vi "Delete Zero.vi"(1 "Unique P-Waves":dbl[](array[numeric])) -> (0 "P-Waves Locations (s)":dbl[](array[numeric]) format="%.2p")   [LabVIEW 2018]
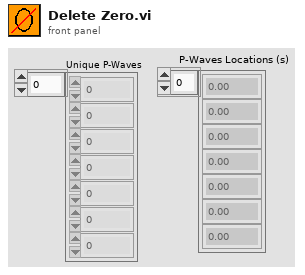
[diagram p1: front panel]
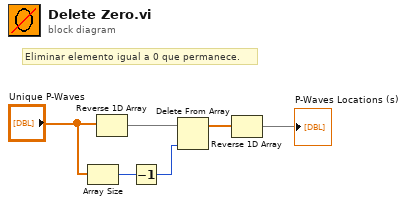
[diagram p0: block diagram]
diagram:
  # "Eliminar elemento igual a 0 que permanece."
  n1 = Array Size(array="Unique P-Waves") -> (size(s)=w4:i32)
  n2 = Reverse 1D Array(array="Unique P-Waves") -> (reversed array=w6:dbl[])
  n3 = Decrement(x=w4) -> (x-1=w3:i32)
  n4 = Delete From Array(array=w6, index=w3) -> (array with subset deleted=w2:dbl[])  [unwired: 1 in, 1 out]
  n5 = Reverse 1D Array(array=w2) -> (reversed array=→"P-Waves Locations (s)":dbl[])
